vi "Parse Lightfield.vi"() -> ()   [LabVIEW 2015]
uses:
  <vilib>/Utility/file.llb/Write Delimited Spreadsheet (string).vi
  <vilib>/Utility/file.llb/Write Delimited Spreadsheet (DBL).vi
  <vilib>/vision/NI_Vision_Development_Module.lvlib
panel:
  in  "Y Coordinate":i32
  in  "X Coordinate":i32
  out "subarray":i64[](array[numeric])
  in  "Filename":string
  in  "Save data":bool
  in  "Calculate":bool=TRUE
  out "Time array":dbl[](array[numeric])
  in  "index (page)":i32
  in  "stop":bool
  out "element":i32=42019
  out "Raw Data":u16[][][](array[numeric])
  in  "length":i32=260
  in  "tf":dbl=0.25
  in  "t0":dbl=930.0
  out "XY Graph":cluster{dbl[], sgl[]}(graph)
  in  "New File":bool=TRUE
  out "selected path":path
  out "Image":T1(plugin-control)
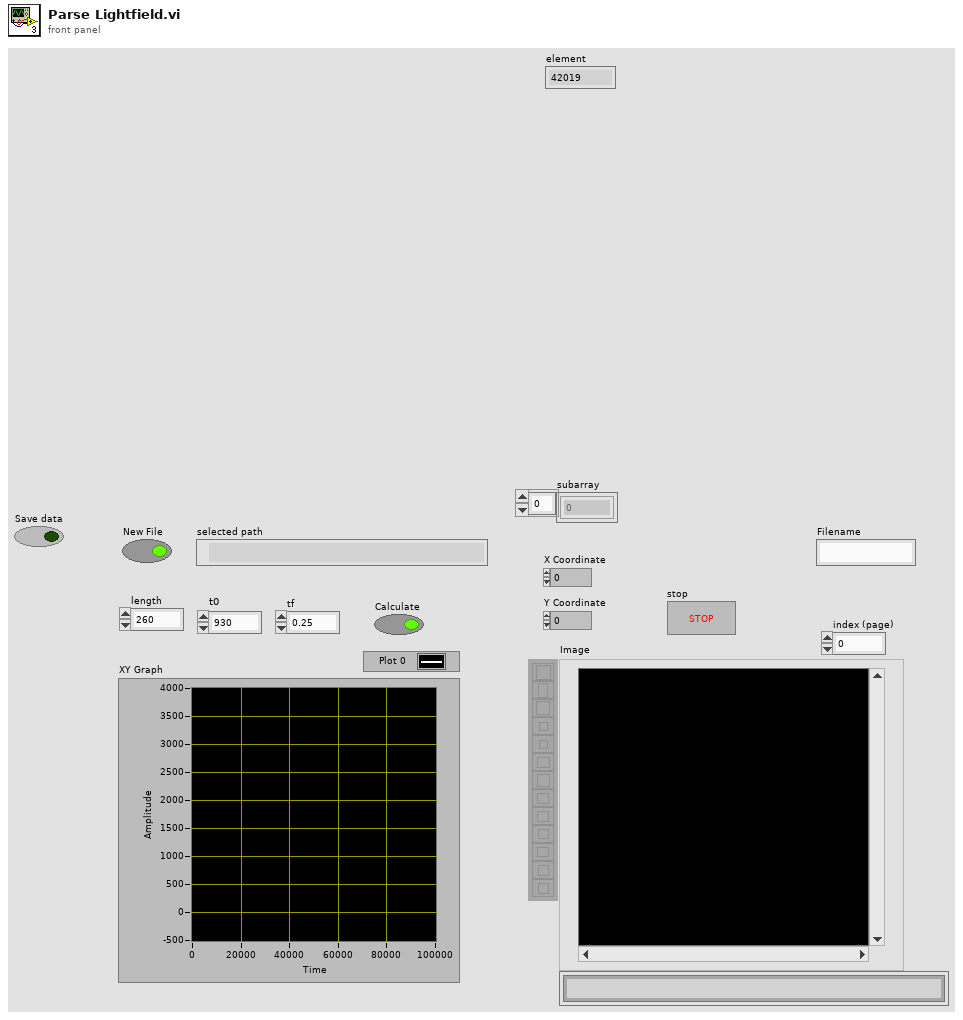
[diagram p1: front panel]
types:
  T1 = typedef "IMAQ Image.ctl" = refnum<image>
  T2 = typedef "Image Type" = u32
  T3 = cluster{"Global Rectangle":i32[], "Contours":cluster{"Contour Type":u32, "ROI Type":u32, "Points":i32[]}[]}
  T4 = cluster{"Mean Value":sgl, "Standard Variation":sgl, "Minimal Value":sgl, "Maximal Value":sgl, "Area (calibrated)":sgl, "Area (pixels)":u32, "%":sgl, "Calibration Valid":bool}
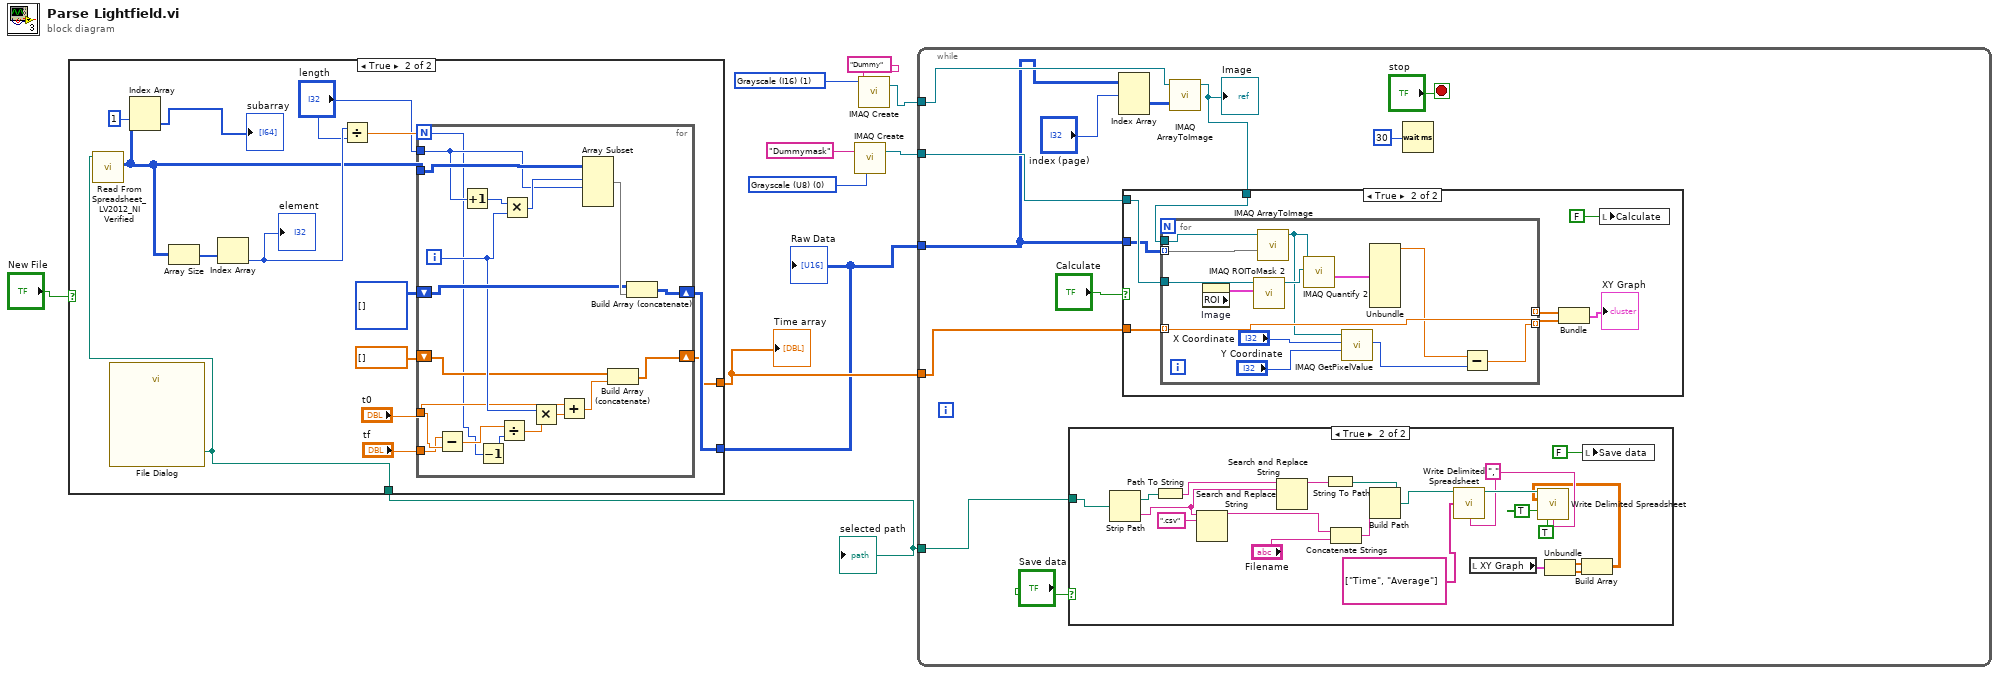
[diagram p0: block diagram]
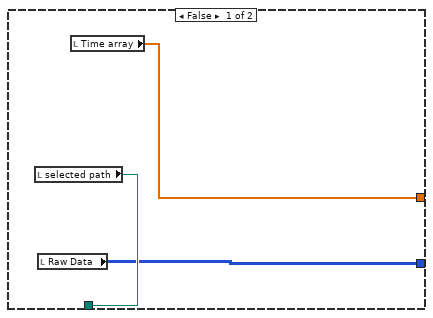
[diagram p4: hidden frame]
diagram:
  w3 = T2 0 items=["Grayscale (U8)", "Grayscale (I16)", "Grayscale (SGL)", "Complex (CSG)", "RGB (U32)", "HSL (U32)", "RGB (U64)", "Grayscale (U16)"] ("Image Type")
  w9 = T2 1 items=["Grayscale (U8)", "Grayscale (I16)", "Grayscale (SGL)", "Complex (CSG)", "RGB (U32)", "HSL (U32)", "RGB (U64)", "Grayscale (U16)"] ("Image Type")
  n1 = case shown="True" "New File" {
    tunnel: [w13 w27] -> w1
    tunnel: [w12 w21] -> w5
    tunnel: [w11 w20] -> w6
    frame False {
      n2 = local read "selected path"() -> (w13:path)
      n3 = local read "Raw Data"() -> (w12:u16[][][])
      n4 = local read "Time array"() -> (w11:dbl[])
    }
    frame True {
      n5 = call "File Dialog"() -> ("selected path"=w27:path)  [unwired: 12 in, 3 out]
      n6 = call "Read From Spreadsheet_LV2012_NI Verified.vi"("Spreadsheet path (.csv)"=w27) -> ("Data Display"=w14:i64[][])  [unwired: 9 in, 1 out]
      n7 = Index Array(array=w14, index (row)=1) -> (element=→"subarray":i64[])  [unwired: 1 in]
      n8 = Array Size(array=w14) -> (size(s)=w23:i32[])
      n9 = Index Array(array=w23) -> (element=w22:i32)  [unwired: 1 in]
      "element" <- w22
      n10 = Divide(x=w22, y="length") -> (x/y=w26:dbl)
      n11 = for {
        N: w26 -> [w29]
        tunnel: w14 -> [w43]
        tunnel: "length" -> [w42]
        shift-right: [w40] -> w21
        shift-left: i64[][][] [] -> [w39]
        shift-right: [w37] -> w20
        shift-left: dbl[] [] -> [w34]
        tunnel: "t0" -> [w31]
        tunnel: "tf" -> [w30]
        i -> [w36]
        n12 = Subtract(x=w30, y=w31) -> (x-y=w32:dbl)
        n13 = Increment(x=w42) -> (x+1=w44:i32)
        n14 = Decrement(x=w29) -> (x-1=w28:i32)
        n15 = Divide(x=w32, y=w28) -> (x/y=w33:dbl)
        n16 = Multiply(x=w44, y=w36) -> (x*y=w45:i32)
        n17 = Multiply(x=w36, y=w33) -> (x*y=w35:dbl)
        n18 = Add(x=w31, y=w35) -> (x+y=w38:dbl)
        n19 = Array Subset(array=w43, index (row)=w45, length (row)=w42) -> (w41:i64[][])  [unwired: 2 in]
        n20 = Build Array (concatenate)(w34, w38) -> (w37:dbl[])
        n21 = Build Array (concatenate)(w39, w41) -> (w40:i64[][][])
      }
    }
  }
  "selected path" <- w1
  "Raw Data" <- w5
  "Time array" <- w6
  n22 = call "IMAQ Create"("Image Name"="Dummymask", "Image Type"=w3) -> ("New Image"=w2:T1)  [unwired: 3 in, 1 out]
  n23 = call "IMAQ Create"("Image Name"="Dummy", "Image Type"=w9) -> ("New Image"=w7:T1)  [unwired: 3 in, 1 out]
  n24 = while {
    tunnel: w5 -> [w52]
    tunnel: w7 -> [w54]
    tunnel: w6 -> [w51]
    tunnel: w2 -> [w53]
    tunnel: w1 -> [w47]
    stop <- "stop" stop-if-true
    n25 = case shown="True" "Save data" {
      tunnel: w47 -> [_ w72]
      frame False {
      }
      frame True {
        w60 = "," ("delimiter (\\t)")
        n26 = Strip Path(path=w72) -> (stripped path=w73:path, name=w67:string)
        n27 = Path To String(path=w73) -> (string=w74:string)
        n28 = Search and Replace String(input string=w67, search string=".csv") -> (result string=w65:string)  [unwired: 6 in, 3 out]
        n29 = Search and Replace String(input string=w74, search string=w67) -> (result string=w75:string)  [unwired: 6 in, 3 out]
        n30 = String To Path(string=w75) -> (path=w69:path)
        n31 = Concatenate Strings(w65, "Filename") -> (w68:string)
        n32 = Build Path(base path=w69, name or relative path=w68) -> (appended path=w63:path)
        n33 = call-poly <vilib>:"Write Delimited Spreadsheet.vi"("file path (dialog if empty)"=w63, "1D data"=string[] ["Time", "Average"], "delimiter (\\t)"=w60) -> ("new file path (Not A Path if cancelled)"=w62:path)  [unwired: 11 in, 1 out]
        n34 = local read "XY Graph"() -> (w78:cluster{dbl[], sgl[]})
        n35 = Unbundle(w78) -> (w77:dbl[], w76:sgl[])
        n36 = Build Array(w77, w76) -> (w58:dbl[][])
        n37 = call-poly <vilib>:"Write Delimited Spreadsheet.vi"("file path (dialog if empty)"=w62, "2D data"=w58, "append to file? (F)"=TRUE, "transpose? (F)"=TRUE, "delimiter (\\t)"=w60) -> ()  [unwired: 9 in, 2 out]
        n38 = local write "Save data"(FALSE ("Save data")) -> ()
      }
    }
    n39 = Index Array(array=w52, index (dim 0)="index (page)") -> (element=w46:i64[][])  [unwired: 2 in]
    n40 = call "IMAQ ArrayToImage"("Image Pixels (I16)"=w46, "Image"=w54) -> ("Image Out"=w50:T1)  [unwired: 8 in, 1 out]
    "Image" <- w50
    n41 = case shown="True" "Calculate" {
      tunnel: w53 -> [_ w83]
      tunnel: w52 -> [_ w82]
      tunnel: w51 -> [_ w81]
      tunnel: w50 -> [_ w80]
      frame False {
      }
      frame True {
        n42 = for {
          tunnel: w82 -> [w93] mode=indexing
          tunnel: w81 -> [w97] mode=indexing
          tunnel: [w97] -> w84 mode=indexing
          tunnel: [w87] -> w85 mode=indexing
          tunnel: w80 -> [w96]
          tunnel: w83 -> [w94]
          n43 = property on="Image" class="ImageControl"() -> ("ROI"=w98:T3)  [unwired: 2 in, 2 out]
          n44 = call "IMAQ ROIToMask 2"("ROI Descriptor"=w98, "Image"=w94) -> ("Image Out"=w95:T1)  [unwired: 7 in, 2 out]
          n45 = call "IMAQ ArrayToImage"("Image Pixels (I16)"=w93, "Image"=w96) -> ("Image Out"=w92:T1)  [unwired: 8 in, 1 out]
          n46 = call "IMAQ Quantify 2"("Image Mask"=w95, "Image"=w92) -> ("Global Report"=w99:T4)  [unwired: 7 in, 2 out]
          n47 = call "IMAQ GetPixelValue"("Image"=w92, "X Coordinate"="X Coordinate", "Y Coordinate"="Y Coordinate") -> ("Pixel Value (I16)"=w89:i16)  [unwired: 3 in, 4 out]
          n48 = Unbundle(w99) -> ("Mean Value"=w88:sgl)  [unwired: 7 out]
          n49 = Subtract(x=w88, y=w89) -> (x-y=w87:sgl)
        }
        n50 = Bundle(w84, w85) -> (→"XY Graph":cluster{dbl[], sgl[]})  [unwired: 1 in]
        n51 = local write "Calculate"(FALSE ("Calculate")) -> ()
      }
    }
    n52 = Wait (ms)(milliseconds to wait=u32 30) -> ()  [unwired: 1 out]
  }
